vi "Run.vi"(8 "error in (no error)":errorcluster, 11 "Opctics in":refnum<class "Opt_Selector.lvclass">) -> (0 "error out":errorcluster, 3 "Opt_Selector out":refnum<class "Opt_Selector.lvclass">)   [LabVIEW 2018, in "Opt_Selector.lvclass"]
uses:
  Opt_Selector.lvclass
  C:/Users/observer/Desktop/Sparc4GUI/SPARC4_GUI/Device/Optics/Optics.lvclass
  Optics.lvclass/Optics.ctl
  Optics.lvclass
  StateMachine/State Machine.lvclass
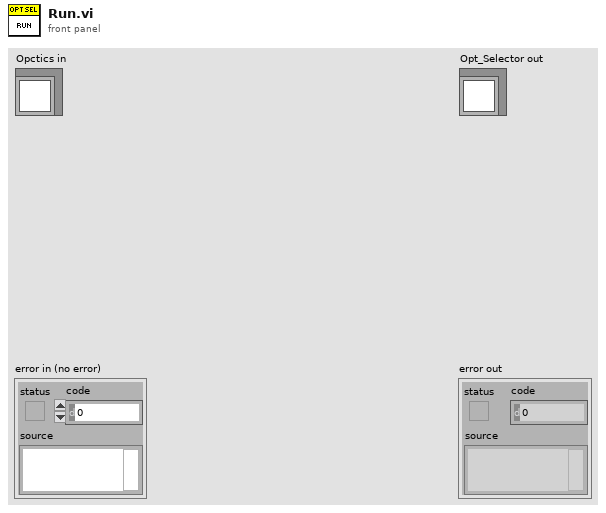
[diagram p1: front panel]
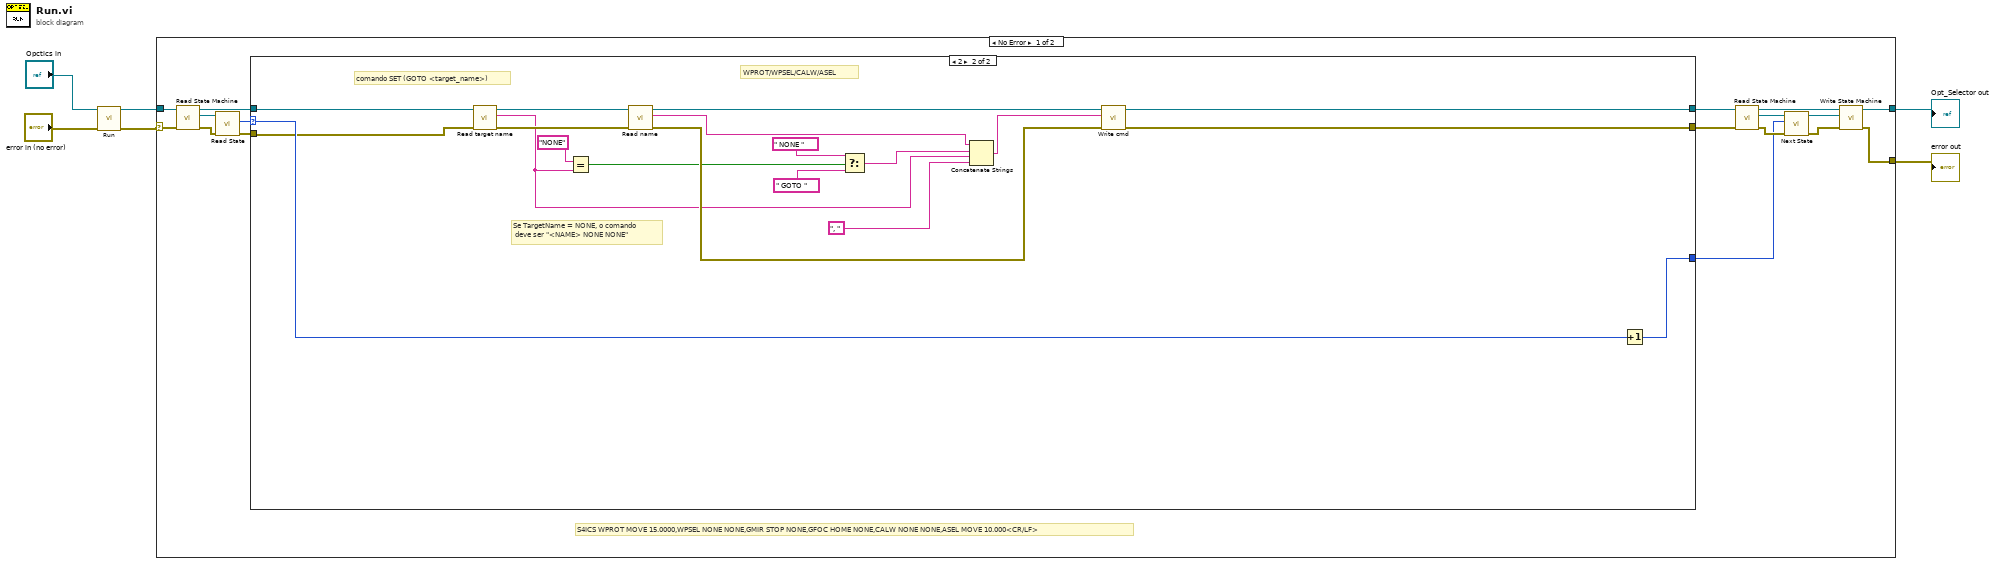
[diagram p0: block diagram]
diagram:
  n1 = call-parent "Run.vi"("error in (no error)"="error in (no error)", "Opctics in"="Opctics in") -> ("error out"=w3:errorcluster, "Optics out"=w4:refnum<class "Opt_Selector.lvclass">)  [unwired: 8 in]
  n2 = case shown="No Error" w3 {
    selector: w3 -> [w22 w47]
    tunnel: [w7 w47] -> w1
    tunnel: [w12 w46] -> w2
    tunnel: w4 -> [w23 w46]
    frame No Error {
      # "S4ICS WPROT MOVE 15.0000,WPSEL NONE NONE,GMIR STOP NONE,GFOC HOME NONE,CALW NONE NONE,ASEL MOVE 10.000<CR/LF>"
      n3 = call-dynamic "Read State Machine.vi"("error in (no error)"=w22, "Device in"=w23) -> ("error out"=w19:errorcluster, "State Machine.lvclass"=w21:refnum<class "State Machine.lvclass">, "Device out"=w17:refnum<class "Opt_Selector.lvclass">)  [unwired: 7 in]
      n4 = call-dynamic "Read State.vi"("error in (no error)"=w19, "State Machine in"=w21) -> ("error out"=w18:errorcluster, "State"=w20:i32)  [unwired: 7 in, 1 out]
      n5 = case shown="2" w20 {
        selector: w20 -> [w26 w41]
        tunnel: w18 -> [w24 w39]
        tunnel: [w24 w44] -> w8
        tunnel: w17 -> [w25 w40]
        tunnel: [w25 w45] -> w15
        tunnel: [w26 w42] -> w9
        frame Default {
        }
        frame 2 {
          # "Se TargetName = NONE, o comando\n deve ser \"<NAME> NONE NONE\""
          # "WPROT/WPSEL/CALW/ASEL"
          # "comando SET (GOTO <target_name>)"
          n6 = call "Read target name.vi"("error in (no error)"=w39, "Optics in"=w40) -> ("error out"=w37:errorcluster, "target name"=w31:string, "Optics out"=w35:refnum<class "Opt_Selector.lvclass">)  [unwired: 7 in]
          n7 = Equal?(x="NONE" ("y"), y=w31) -> (x = y?=w32:bool)
          n8 = call "Read name.vi"("error in (no error)"=w37, "Optics in"=w35) -> ("error out"=w36:errorcluster, "name"=w38:string, "Optics out"=w34:refnum<class "Opt_Selector.lvclass">)  [unwired: 7 in]
          n9 = Select(t=" NONE " ("string"), s=w32, f=" GOTO " ("string")) -> (s? t:f=w28:string)
          n10 = Concatenate Strings(w38, w28, w31, ", ") -> (w43:string)
          n11 = call-dynamic "Write cmd.vi"("error in (no error)"=w36, "cmd"=w43, "Device in"=w34) -> ("error out"=w44:errorcluster, "Device out"=w45:refnum<class "Opt_Selector.lvclass">)  [unwired: 7 in]
          n12 = Increment(x=w41) -> (x+1=w42:i32)
        }
      }
      n13 = call-dynamic "Read State Machine.vi"("error in (no error)"=w8, "Device in"=w15) -> ("error out"=w11:errorcluster, "State Machine.lvclass"=w14:refnum<class "State Machine.lvclass">, "Device out"=w13:refnum<class "Opt_Selector.lvclass">)  [unwired: 7 in]
      n14 = call "Next State.vi"("error in (no error)"=w11, "New_State"=w9, "State Machine in"=w14) -> ("error out"=w10:errorcluster, "State Machine out"=w16:refnum<class "State Machine.lvclass">)  [unwired: 7 in]
      n15 = call-dynamic "Write State Machine.vi"("error in (no error)"=w10, "State Machine.lvclass"=w16, "Device in"=w13) -> ("error out"=w7:errorcluster, "Device out"=w12:refnum<class "Opt_Selector.lvclass">)  [unwired: 7 in]
    }
    frame Error {
    }
  }
  "error out" <- w1
  "Opt_Selector out" <- w2
